vi "P3.vi"(1 "C2":waveform(dbl)={"t0"=timestamp(0 s since 1904-01-01), "dt"=0.0, "Y"=[]}, 2 "C1":waveform(dbl)={"t0"=timestamp(0 s since 1904-01-01), "dt"=0.0, "Y"=[]}) -> (0 "CO":waveform(dbl))   [LabVIEW 2010]
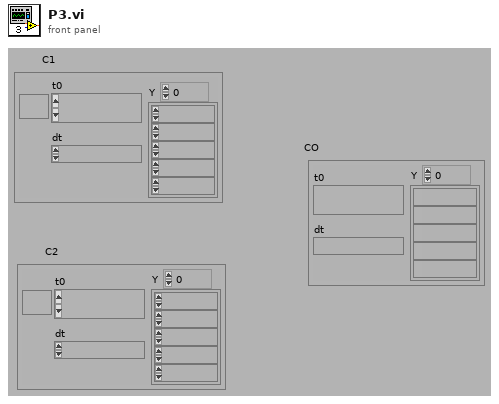
[diagram p1: front panel]
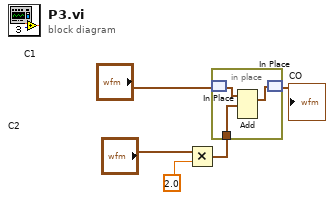
[diagram p0: block diagram]
diagram:
  n1 = Multiply(x="C2", y=2.0) -> (x*y=w4:waveform(dbl))
  n2 = in-place {
    in-place-border: w4 -> [w8]
    n3 = in-place-match #1("C1") -> (w7:waveform(dbl))
    n4 = Add(1:w8, 2:w7) -> (0:w6:waveform(dbl))  [unwired: 1 in, 1 out]
    n5 = in-place-match #1(w6) -> (→"CO":waveform(dbl))
  }
